vi "2B_Tech Serial Data Recording & DECADE 2.0.vi"() -> ()   [LabVIEW 2014]
uses:
  <vilib>/Instr/_visa.llb/VISA Set IO Buffer Mask.ctl
  <vilib>/Instr/_visa.llb/VISA Flush IO Buffer Mask.ctl
  <vilib>/Platform/TimedLoop/XDataNode/timing_clust.ctl
  <vilib>/Platform/TimedLoop/XDataNode/nitl_modes.ctl
  <vilib>/Platform/TimedLoop/XDataNode/wakeup.ctl
  C:/Program Files (x86)/National Instruments/LabVIEW 2014/examples/Data Communication/Network Streams/Simple Network Streams/support/Network Stream Command.ctl
  <vilib>/Utility/error.llb/whitespace.ctl
  <vilib>/Instr/_visa.llb/VISA Configure Serial Port (Instr).vi
  <vilib>/Utility/tcp.llb/UDP Multicast Write-Only Open.vi
  <vilib>/platform/TimedLoop/XDataNode/XDataNode.xnode
  <vilib>/Platform/TimedLoop/XDataNode/XDNodeRunTimeDep.lvlib
panel:
  out "Default file name":string
  out "error out":errorcluster
  out "Ambient/Cabin":bool
  out "Stop File Write":bool
  in  "timeout (10sec)":u32=3000
  in  "VISA resource name":refnum<visa-resource-name>="ASRL2::INSTR"
  out "Simulate 3 av":dbl
  out "Simulate\nConc":i32
  out "Simulate\nconc":bool
  out "3hr_alm_thresh":i32=80
  out "3hrAvg_Alarm":bool
  out "Inst_Alarm":bool
  out "Inst_alm_thresh":i32=220
  out "Time":string
  in  "Clear Display\nErrors":bool
  out "Read Error Counter\nfrom process loop":u32
  out "CABOZO UDP_ASCII_Out":string
  out "Ozo_array":string[](array[string])
  out "3hr_ozo_avg":dbl
  out "q_size":i32
  out "Data Output":string[](array[string])
  out "UDP packet\nSend status":bool
  out "TWBOZO UDP_ASCII_Out":string
  out "UDP_Out_Error":errorcluster
  out "UDP_Pack_num":u32
  out "Flight Number":string
  out "Number of times \nRead time out":u32
  out "Data Loop count":i32
  out "2B_Serial_error out":errorcluster
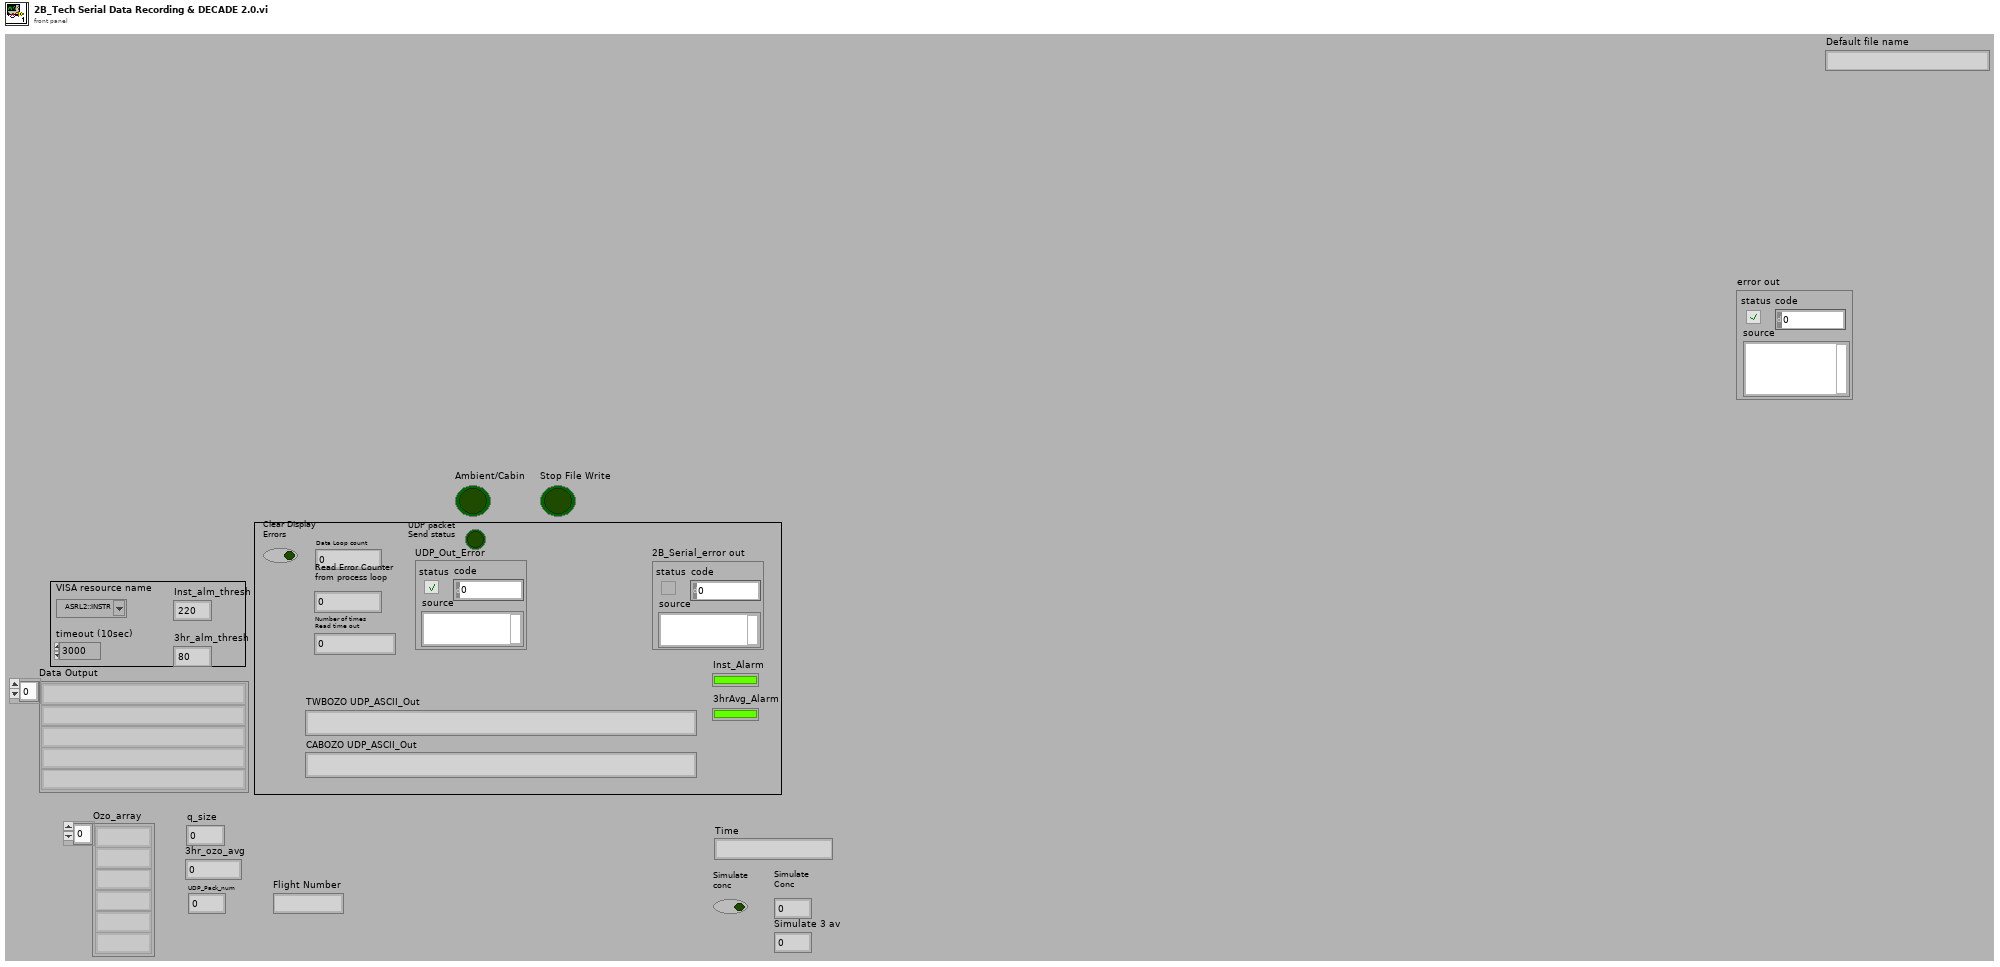
[diagram p1: front panel]
types:
  T1 = typedef "VISA Flush IO Buffer Mask.ctl" = u16
  T2 = typedef "VISA Set IO Buffer Mask.ctl" = u16
  T3 = typedef "Network Stream Command.ctl" = cluster{"Message":string, "Message Data":variant}
  T4 = typedef "XDNodeRunTimeDep.lvlib/timing_clust.ctl" = cluster{"Expected End [f-1]":u64, "Actual End [f-1]":u64, "Finished Late? [f-1]":bool, "Expected End [i-1]":u64, "Actual End [i-1]":u64, "Finished Late? [i-1]":bool, "Expected Start [i]":u64, "Actual Start [i]":u64, "Expected Start [f]":u64, "Actual Start [f]":u64, "Source Name":string, "Structure Name":string, "Period":i64, "Deadline":i64, "Offset":i64, "Start":i64, "Priority":i32, "Timeout":i32, "Mode":T5, "Wakeup Reason":T6, "Error":errorcluster, "Source Type":string, "Secondary Source Type":string, "Global End Time":u64, "Global Start Time":u64, "Frame Duration":u64, "Iteration Duration":u64, "Assigned CPU":i32, "I/O Scan Engine Mode":u32}
  T5 = typedef "XDNodeRunTimeDep.lvlib/nitl_modes.ctl" = enum32{"No Change", "Process missed periods, maintain original phase", "Discard missed periods, maintain original phase", "Process missed periods, ignore original phase", "Discard missed periods, ignore original phase"}
  T6 = typedef "XDNodeRunTimeDep.lvlib/wakeup.ctl" = enum32{"Normal", "Aborted", "Asynchronous wakeup", "Timing source error", "Timed loop error", "Timeout"}
  T7 = enum16{"open", "replace", "create", "open or create", "replace or create", "replace or create with confirmation"}
  T8 = typedef "whitespace.ctl" = u16
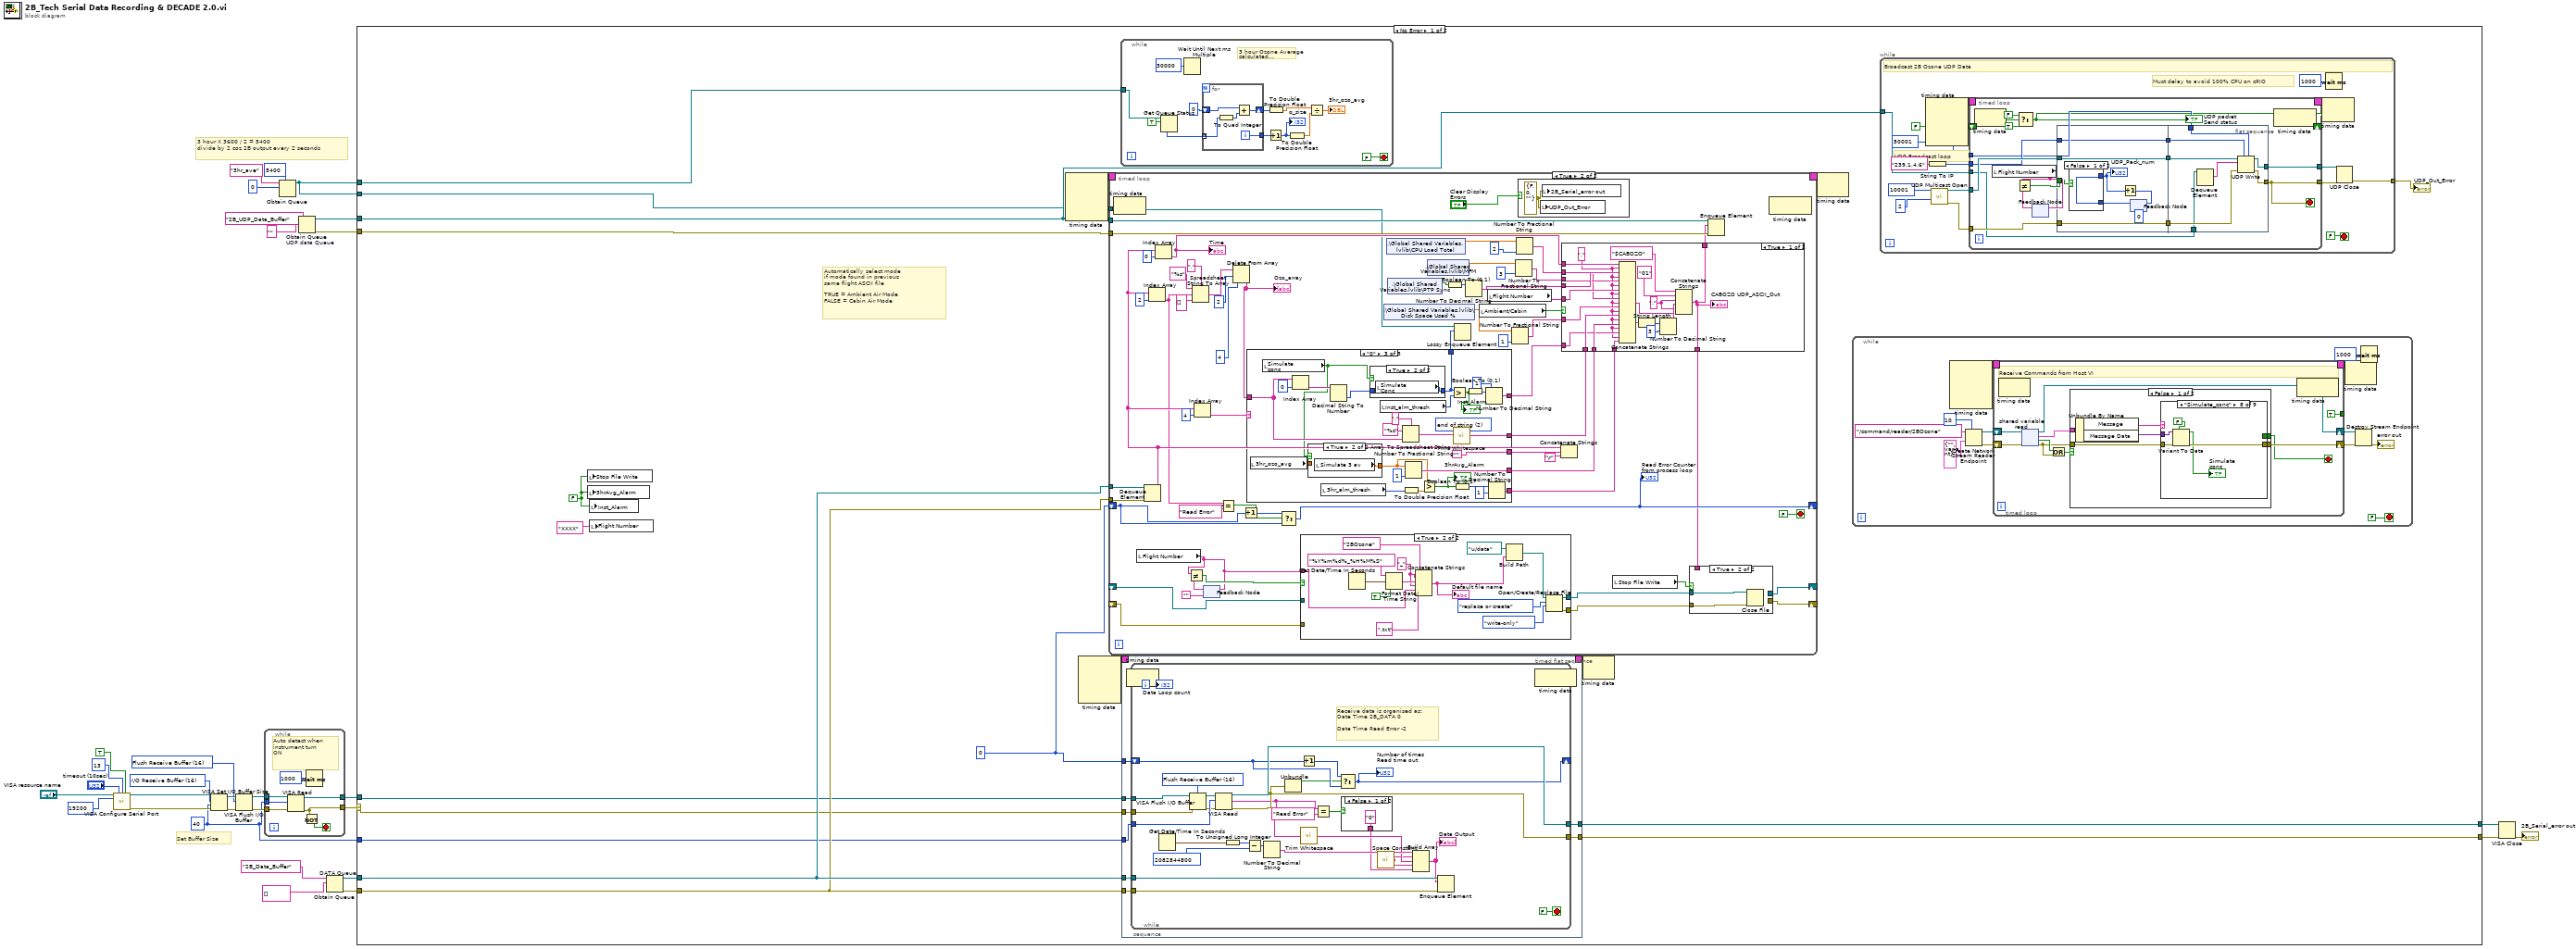
[diagram p0: block diagram]
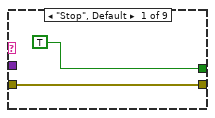
[diagram p2: hidden frame]
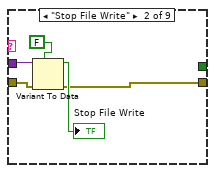
[diagram p3: hidden frame]
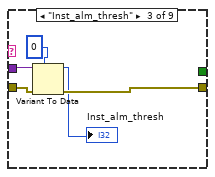
[diagram p4: hidden frame]
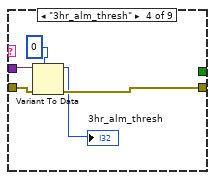
[diagram p5: hidden frame]
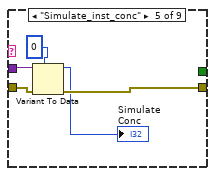
[diagram p6: hidden frame]
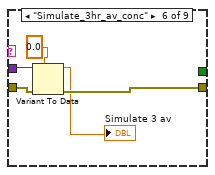
[diagram p7: hidden frame]
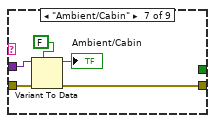
[diagram p8: hidden frame]
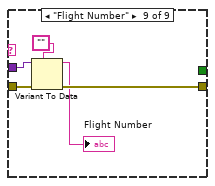
[diagram p9: hidden frame]
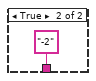
[diagram p11: hidden frame]
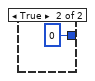
[diagram p12: hidden frame]
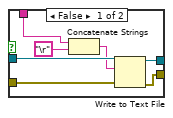
[diagram p13: hidden frame]
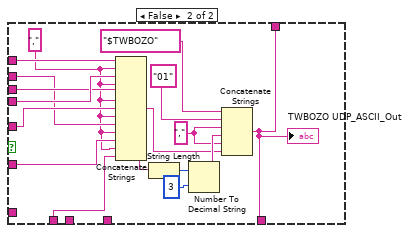
[diagram p16: hidden frame]
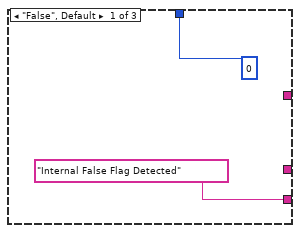
[diagram p17: hidden frame]
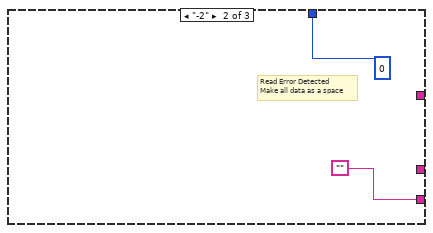
[diagram p18: hidden frame]
diagram:
  w1 = u32 40 ("size (4096)")
  w8 = T1 16 items=["Flush Receive Buffer"=16, "Write Transmit Buffer to Device"=32, "Flush Receive Buffer (No I/O)"=64, "Flush Transmit Buffer"=128] ("Mask")
  w9 = T2 16 items=["I/O Receive Buffer"=16, "I/O Transmit Buffer"=32, "I/O Receive and Transmit Buffer"=48] ("Mask")
  # "Set Buffer Size"
  # "3 hour X 3600 / 2 = 5400\ndivide by 2 coz 2B output every 2 seconds"
  n1 = call-poly "VISA Configure Serial Port"("VISA resource name"="VISA resource name", "timeout (10sec)"="timeout (10sec)", "termination char\n(0xA = '\\n' = LF)"=u8 13 ("termination char\n(0xA = '\\n' = LF)"), "Enable Termination\nChar (T)"=TRUE ("Enable Termination\nChar (T)"), "baud rate (9600)"=u32 19200) -> ("VISA resource name out"=w7:refnum<visa-resource-name>, "error out"=w6:errorcluster)  [unwired: 9 in]
  n2 = VISA Set I/O Buffer Size(VISA resource name=w7, mask (16)=w9, size (4096)=w1, error in (no error)=w6) -> (VISA resource name out=w10:refnum<visa-resource-name>, error out=w11:errorcluster)
  n3 = VISA Flush I/O Buffer(VISA resource name=w10, mask (16)=w8, error in (no error)=w11) -> (VISA resource name out=w5:refnum<visa-resource-name>, error out=w4:errorcluster)
  n4 = while {
    tunnel: w1 -> [w38]
    tunnel: w5 -> [w37]
    tunnel: w4 -> [w36]
    tunnel: [w34] -> w3
    tunnel: [w33] -> w2
    stop <- w35 stop-if-true
    # "Auto detect when\ninstrument turn\nON"
    n5 = VISA Read(VISA resource name=w37, byte count=w38, error in (no error)=w36) -> (VISA resource name out=w33:refnum<visa-resource-name>, error out=w34:errorcluster)  [unwired: 2 out]
    n6 = Not(x=w34) -> (.not. x?=w35:bool)
    n7 = Wait (ms)(milliseconds to wait=u32 1000) -> ()  [unwired: 1 out]
  }
  n8 = Obtain Queue(max queue size (-1, unlimited)=5400, name (unnamed)="3hr_ave", element data type=0 ("index")) -> (queue out=w17:refnum<queue>)  [unwired: 2 in, 2 out]
  n9 = Obtain Queue "UDP data Queue"(name (unnamed)="2B_UDP_Data_Buffer", element data type="") -> (queue out=w23:refnum<queue>, error out=w22:errorcluster)  [unwired: 3 in, 1 out]
  n10 = Obtain Queue "DATA Queue"(name (unnamed)="2B_Data_Buffer", element data type=string[] []) -> (queue out=w27:refnum<queue>, error out=w26:errorcluster)  [unwired: 3 in, 1 out]
  n11 = case shown="No Error" w3 {
    selector: w3 -> [w44 w417]
    tunnel: w2 -> [w45 w418]
    tunnel: [w57 w418] -> w30
    tunnel: [w49 w417] -> w31
    tunnel: w27 -> [w56 _]
    tunnel: w26 -> [w55 _]
    tunnel: w23 -> [w53 _]
    tunnel: w22 -> [w54 _]
    tunnel: w17 -> [w52 _]
    tunnel: w17 -> [w51 _]
    tunnel: w1 -> [w43 _]
    frame No Error {
      w40 = FALSE
      w50 = u32 0
      # "Automatically select mode\nif mode found in previous\nsame flight ASCII file\n\nTRUE = Ambient Air Mode\nFALSE = Cabin Air Mode"
      n12 = local write "Stop File Write"(w40) -> ()
      n13 = local write "3hrAvg_Alarm"(w40) -> ()
      n14 = local write "Inst_Alarm"(w40) -> ()
      n15 = local write "Flight Number"("XXXX" ("Flight Number")) -> ()
      n16 = node-c288() -> (w48:T4)  [unwired: 4 in]
      n17 = node-c288() -> (w42:T4)  [unwired: 4 in]
      n18 = timed-loop {
        timing: w48 -> [_]
        timing-out: [_] -> w47
        tunnel: w56 -> [w315]
        tunnel: w55 -> [w314]
        tunnel: w53 -> [w313]
        tunnel: w54 -> [w312]
        tunnel: w51 -> [w284]
        shift-right: [w288] -> _
        shift-left: w50 -> [w289]
        shift-right: [w277] -> _
        shift-left: _ -> [w273]
        shift-right: [w271] -> _
        shift-left: _ -> [w272]
        stop <- FALSE stop-if-true
        n19 = node-c288() -> ()  [unwired: 1 in, 1 out]
        n20 = local read "Flight Number"() -> (w269:string)
        n21 = Dequeue Element(queue=w315, error in (no error)=w314) -> (element=w297:string[])  [unwired: 1 in, 3 out]
        n22 = Index Array(array=w297, index=2) -> (element=w290:string)
        n23 = Index Array(array=w297, index=0) -> (element=w299:string)
        "Time" <- w299
        n24 = Spreadsheet String To Array(delimiter (Tab)=",", format string="%s", spreadsheet string=w290, array type (2D Dbl)=string[] [] ("Values Array")) -> (array=w304:string[])
        n25 = Index Array(array=w297, index=4) -> (element=w305:string)
        n26 = feedback #1("" ("Flight Number")) -> (w279:string)
        n27 = Not Equal?(x=w269, y=w279) -> (x != y?=w270:bool)
        n28 = feedback-in #1(w269) -> ()
        n29 = Equal?(x=w290, y="Read Error") -> (x = y?=w292:bool)
        n30 = Delete From Array(array=w304, length=2, index=4) -> (array with subset deleted=w301:string[])  [unwired: 1 out]
        "Ozo_array" <- w301
        n31 = Increment(x=w289) -> (x+1=w291:u32)
        n32 = case shown="\"0\"" w305 {
          tunnel: w301 -> [_ _ w401]
          tunnel: [_ _ w404] -> w298
          tunnel: [0 0 w389] -> w283
          tunnel: ["Internal False Flag Detected" "" ""] -> w296
          tunnel: [_ _ w398] -> w294
          tunnel: [_ _ w395] -> w286
          tunnel: [_ _ w391] -> w285
          frame "False", Default {
          }
          frame "-2" {
            # "Read Error Detected\nMake all data as a space"
          }
          frame "0" {
            w405 = T8 2 items=["both", "start of string", "end of string"] ("location (both)")
            n33 = local read "3hr_ozo_avg"() -> (w388:dbl)
            n34 = local read "Simulate\nconc"() -> (w384:bool)
            n35 = Index Array(array=w401, index=0) -> (element=w402:string)
            n36 = case shown="True" w384 {
              tunnel: [w409 w410] -> w387
              tunnel: w388 -> [w409 _]
              frame False {
              }
              frame True {
                n37 = local read "Simulate 3 av"() -> (w410:dbl)
              }
            }
            n38 = local read "3hr_alm_thresh"() -> (w385:i32)
            n39 = Decimal String To Number(string=w402) -> (number=w390:i32)  [unwired: 2 in, 1 out]
            n40 = case shown="True" w384 {
              tunnel: [w411 w412] -> w389
              tunnel: w390 -> [w411 _]
              frame False {
              }
              frame True {
                n41 = local read "Simulate\nConc"() -> (w412:i32)
              }
            }
            n42 = local read "Inst_alm_thresh"() -> (w386:i32)
            n43 = Array To Spreadsheet String(delimiter (Tab)=",", array=w401, 3:"%s" ("format string")) -> (spreadsheet string=w406:string)
            n44 = To Double Precision Float(number=w385) -> (double precision float=w392:dbl)
            n45 = Number To Fractional String(number=w387, precision (6)=i16 1) -> (F-format string=w398:string)  [unwired: 2 in]
            n46 = Greater?(x=w387, y=w392) -> (0:w393:bool)
            "3hrAvg_Alarm" <- w393
            n47 = Greater?(x=w389, y=w386) -> (0:w396:bool)
            "Inst_Alarm" <- w396
            n48 = call <vilib>:"Trim Whitespace.vi"("string"=w406, "location (both)"=w405) -> ("trimmed string"=w404:string)
            n49 = Boolean To (0,1)(Boolean=w393) -> (0, 1=w394:i16)
            n50 = Boolean To (0,1)(Boolean=w396) -> (0, 1=w397:i16)
            n51 = Number To Decimal String(number=w397, width (-)=i16 1) -> (decimal integer string=w395:string)
            n52 = Number To Decimal String(number=w394, width (-)=i16 1) -> (decimal integer string=w391:string)
          }
        }
        n53 = Select(t=w291, s=w292, f=w289) -> (s? t:f=w288:u32)
        "Read Error Counter\nfrom process loop" <- w288
        n54 = case shown="True" w270 {
          tunnel: [w326 w329] -> w275
          tunnel: [w325 w328] -> w274
          tunnel: w273 -> [w326 _]
          tunnel: w272 -> [w325 _]
          tunnel: w269 -> [_ w327]
          frame False {
          }
          frame True {
            w336 = "_" ("string")
            n55 = Get Date/Time In Seconds() -> (seconds since 1Jan1904=w337:timestamp)
            n56 = Format Date/Time String(time format string (%c)="%Y%m%d%_%H%M%S", seconds (now)=w337, UTC format=TRUE) -> (date/time string=w340:string)
            n57 = Concatenate Strings("2BOzone" ("string"), w336, w340, w336, w327, ".txt" ("string")) -> (w334:string)
            "Default file name" <- w334
            n58 = Build Path(base path=path "u:/data", name or relative path=w334) -> (appended path=w330:path)
            n59 = Open/Create/Replace File(file path (use dialog)=w330, operation (0:open)=T7."replace or create", access (0:read/write)=enum16{"read/write", "read-only", "write-only"}."write-only") -> (refnum out=w329:refnum<file>, error out=w328:errorcluster)  [unwired: 3 in, 1 out]
          }
        }
        n60 = shared-variable ".\\Global Shared Variables.lvlib\\Disk Space Used %"() -> (w257:dbl)  [unwired: 1 in, 1 out]
        n61 = shared-variable ".\\Global Shared Variables.lvlib\\CPU Load Total"() -> (w267:dbl)  [unwired: 1 in, 1 out]
        n62 = shared-variable ".\\Global Shared Variables.lvlib\\PTP Sync"() -> (w260:bool)  [unwired: 1 in, 1 out]
        n63 = shared-variable ".\\Global Shared Variables.lvlib\\MFM"() -> (w265:dbl)  [unwired: 1 in, 1 out]
        n64 = Boolean To (0,1)(Boolean=w260) -> (0, 1=w261:i16)
        n65 = Lossy Enqueue Element(queue=w284, element=w283) -> ()  [unwired: 1 in, 4 out]
        n66 = Number To Decimal String(number=w261) -> (decimal integer string=w259:string)  [unwired: 1 in]
        n67 = local read "Ambient/Cabin"() -> (w280:bool)
        n68 = local read "Flight Number"() -> (w281:string)
        n69 = Number To Fractional String(number=w257, precision (6)=i16 1) -> (F-format string=w256:string)  [unwired: 2 in]
        n70 = Number To Fractional String(number=w265, precision (6)=i16 3) -> (F-format string=w262:string)  [unwired: 2 in]
        n71 = Number To Fractional String(number=w267, precision (6)=i16 2) -> (F-format string=w266:string)  [unwired: 2 in]
        n72 = case shown="True" "Clear Display\nErrors" {
          frame False {
          }
          frame True {
            w342 = errorcluster {"status"=FALSE, "code"=0, "source"=""} ("UDP Error Out")
            n73 = local write "UDP_Out_Error"(w342) -> ()
            n74 = local write "2B_Serial_error out"(w342) -> ()
          }
        }
        n75 = Concatenate Strings(w297, w296, "\r") -> ()  [unwired: 1 out]
        n76 = case shown="True" w280 {
          tunnel: [w349 w369] -> w311
          tunnel: w299 -> [w354 w370]
          tunnel: w298 -> [w353 w362]
          tunnel: w266 -> [w345 w365]
          tunnel: w262 -> [w347 w367]
          tunnel: w281 -> [w346 w366]
          tunnel: w294 -> [w352 _]
          tunnel: w286 -> [w351 _]
          tunnel: w285 -> [w350 _]
          tunnel: [w349 w369] -> w268
          tunnel: w259 -> [w348 w368]
          tunnel: w256 -> [w344 w364]
          frame True {
            w343 = ","
            w358 = ","
            n77 = Concatenate Strings(w354, w343, w348, w343, w347, w343, w346, w343, w345, w343, w344, w343, w353, w343, w352, w343, w351, w343, w350) -> (w357:string)
            n78 = String Length(string=w357) -> (length=w361:i32)
            n79 = Number To Decimal String(number=w361, width (-)=i16 3) -> (decimal integer string=w359:string)
            n80 = Concatenate Strings("$CABOZO", "01", w358, w359, w358, w357) -> (w349:string)
            "CABOZO UDP_ASCII_Out" <- w349
          }
          frame False {
            w363 = ","
            w374 = ","
            n81 = Concatenate Strings(w370, w363, w368, w363, w367, w363, w366, w363, w365, w363, w364, w363, w362) -> (w373:string)
            n82 = String Length(string=w373) -> (length=w377:i32)
            n83 = Number To Decimal String(number=w377, width (-)=i16 3) -> (decimal integer string=w375:string)
            n84 = Concatenate Strings("$TWBOZO", "01", w374, w375, w374, w373) -> (w369:string)
            "TWBOZO UDP_ASCII_Out" <- w369
          }
        }
        n85 = local read "Stop File Write"() -> (w276:bool)
        n86 = case shown="True" w276 {
          tunnel: w275 -> [w322 w324]
          tunnel: w274 -> [w321 w323]
          tunnel: [w318 _] -> w277
          tunnel: [w317 _] -> w271
          tunnel: w268 -> [w316 _]
          frame False {
            n87 = Concatenate Strings(w316, "\r") -> (w319:string)
            n88 = Write to Text File(file (use dialog)=w322, text=w319, error in=w321) -> (refnum out=w318:refnum<file>, error out=w317:errorcluster)  [unwired: 2 out]
          }
          frame True {
            n89 = Close File(refnum=w324, error in=w323) -> ()  [unwired: 2 out]
          }
        }
        n90 = Enqueue Element(queue=w313, element=w311, error in (no error)=w312) -> ()  [unwired: 1 in, 3 out]
        n91 = node-c288() -> ()  [unwired: 1 in, 1 out]
      }
      n92 = while {
        tunnel: w52 -> [w188]
        stop <- FALSE stop-if-true
        # "3 hour Ozone Average calculated\nevery 30 seconds"
        n93 = Get Queue Status(queue=w188, return elements? (F)=TRUE) -> (elements=w185:i32[])  [unwired: 1 in, 7 out]
        n94 = Wait Until Next ms Multiple(millisecond multiple=u32 30000) -> ()  [unwired: 1 out]
        n95 = for {
          tunnel: [w200] -> w195
          shift-right: [w199] -> w193
          shift-left: i64 0 -> [w198]
          tunnel: w185 -> [w196] mode=indexing
          i -> [w200]
          n96 = To Quad Integer(1:w196) -> (0:w197:i64)
          n97 = Add(x=w198, y=w197) -> (x+y=w199:i64)
        }
        n98 = Increment(x=w195) -> (x+1=w189:i32)
        "q_size" <- w189
        n99 = To Double Precision Float(number=w193) -> (double precision float=w191:dbl)
        n100 = To Double Precision Float(number=w189) -> (double precision float=w192:dbl)
        n101 = Divide(x=w191, y=w192) -> (x/y=→"3hr_ozo_avg":dbl)
      }
      n102 = timed-sequence {
        timing: w42 -> [_]
        timing-out: [_] -> w41
        tunnel: [w141] -> w57
        tunnel: w56 -> [w140]
        tunnel: w55 -> [w139]
        tunnel: w50 -> [w138]
        tunnel: [w137] -> w49
        tunnel: w45 -> [w136]
        tunnel: w44 -> [w135]
        tunnel: w43 -> [w134]
        n103 = timed-flat-sequence {
          tunnel: [w149] -> w141
          tunnel: w140 -> [w148]
          tunnel: w139 -> [w147]
          tunnel: w138 -> [w146]
          tunnel: [w145] -> w137
          tunnel: w136 -> [w144]
          tunnel: w135 -> [w143]
          tunnel: w134 -> [w142]
          n104 = node-c288() -> ()  [unwired: 1 in, 1 out]
          n105 = while {
            tunnel: [w168] -> w145
            shift-right: [w174] -> _
            shift-left: w146 -> [w175]
            tunnel: [w177] -> w149
            tunnel: w144 -> [w173]
            tunnel: w143 -> [w172]
            tunnel: w148 -> [w171]
            tunnel: w147 -> [w170]
            tunnel: w142 -> [w169]
            i -> [w176]
            stop <- FALSE stop-if-true
            w153 = T1 16 items=["Flush Receive Buffer"=16, "Write Transmit Buffer to Device"=32, "Flush Receive Buffer (No I/O)"=64, "Flush Transmit Buffer"=128] ("Mask")
            # "Receive data is organised as:\nDate Time 2B_DATA 0\n\nDate Time Read Error -2"
            n106 = Get Date/Time In Seconds() -> (seconds since 1Jan1904=w163:timestamp)
            n107 = VISA Flush I/O Buffer(VISA resource name=w173, mask (16)=w153, error in (no error)=w172) -> (VISA resource name out=w154:refnum<visa-resource-name>, error out=w152:errorcluster)
            n108 = VISA Read(VISA resource name=w154, byte count=w169, error in (no error)=w152) -> (VISA resource name out=w177:refnum<visa-resource-name>, read buffer=w151:string, error out=w168:errorcluster)  [unwired: 1 out]
            n109 = To Unsigned Long Integer(number=w163) -> (unsigned 32bit integer=w165:u32)
            n110 = Subtract(x=w165, y=u32 2082844800) -> (x-y=w162:u32)
            n111 = Number To Decimal String(number=w162) -> (decimal integer string=w159:string)  [unwired: 1 in]
            n112 = Unbundle(w168) -> ("status"=w166:bool)  [unwired: 2 out]
            n113 = Increment(x=w175) -> (x+1=w167:u32)
            n114 = call <vilib>:"Trim Whitespace.vi"("string"=w151) -> ("trimmed string"=w158:string)  [unwired: 1 in]
            n115 = Equal?(x=w151, y="Read Error") -> (x = y?=w160:bool)
            n116 = Select(t=w167, s=w166, f=w175) -> (s? t:f=w174:u32)
            "Number of times \nRead time out" <- w174
            n117 = case shown="False" w160 {
              tunnel: ["0" "-2"] -> w156
              frame False {
              }
              frame True {
              }
            }
            n118 = call <vilib>:"Space Constant.vi"() -> ("String"=w157:string)
            n119 = Build Array(w159, w157, w158, w157, w156) -> (w155:string[])
            "Data Output" <- w155
            n120 = Enqueue Element(queue=w171, element=w155, error in (no error)=w170) -> ()  [unwired: 1 in, 3 out]
            "Data Loop count" <- w176
          }
          n121 = node-c288() -> ()  [unwired: 1 in, 1 out]
        }
      }
      n122 = node-c288(w41) -> ()  [unwired: 1 out]
      n123 = node-c288(w47) -> ()  [unwired: 1 out]
      n124 = while {
        stop <- FALSE stop-if-true
        n125 = node-c288() -> (w59:T4)  [unwired: 4 in]
        n126 = Create Network Stream Reader Endpoint(7:10 ("reader buffer size"), 9:T3 {"Message"="", "Message Data"=variant} ("Message Cluster"), 11:"/command/reader/2BOzone" ("reader url")) -> (0:w65:errorcluster, 3:w66:refnum<k21>)  [unwired: 4 in]
        n127 = timed-loop "Host->Target Command Reader" {
          shift-right: [w76] -> w63
          shift-left: w65 -> [w79]
          shift-right: [w77] -> w62
          shift-left: w66 -> [w78]
          tunnel: [TRUE] -> _
          timing: w59 -> [_]
          timing-out: [_] -> w58
          stop <- w70 stop-if-true
          # "Receive Commands from Host VI"
          n128 = node-c288() -> ()  [unwired: 1 in, 1 out]
          n129 = shared-variable-read(w78, w79) -> (w77:refnum<k21>, w72:errorcluster, w74:bool, w75:T3)  [unwired: 1 in]
          n130 = Or(x=w74, y=w72) -> (x .or. y?=w73:bool)
          n131 = case shown="False" w73 {
            selector: w73 -> [_ w130]
            tunnel: w72 -> [w87 w131]
            tunnel: [w86 w131] -> w76
            tunnel: w75 -> [w84 _]
            tunnel: [w85 w130] -> w70
            frame False {
              n132 = Unbundle By Name(w84) -> ("Message"=w83:string, "Message Data"=w82:variant)
              n133 = case shown="\"Simulate_conc\"" w83 {
                tunnel: w87 -> [w89 w94 w99 w104 w109 w114 w119 w124 w129]
                tunnel: [w89 w90 w97 w102 w107 w112 w118 w123 w128] -> w86
                tunnel: w82 -> [_ w93 w98 w103 w108 w113 w117 w122 w127]
                tunnel: [TRUE _ _ _ _ _ _ _ _] -> w85
                frame "Stop", Default {
                }
                frame "Stop File Write" {
                  n134 = Variant To Data(error in=w94, type=FALSE, Variant=w93) -> (data=→"Stop File Write":bool, error out=w90:errorcluster)
                }
                frame "Inst_alm_thresh" {
                  n135 = Variant To Data(error in=w99, type=0, Variant=w98) -> (data=→"Inst_alm_thresh":i32, error out=w97:errorcluster)
                }
                frame "3hr_alm_thresh" {
                  n136 = Variant To Data(error in=w104, type=0, Variant=w103) -> (data=→"3hr_alm_thresh":i32, error out=w102:errorcluster)
                }
                frame "Simulate_inst_conc" {
                  n137 = Variant To Data(error in=w109, type=0, Variant=w108) -> (data=→"Simulate\nConc":i32, error out=w107:errorcluster)
                }
                frame "Simulate_3hr_av_conc" {
                  n138 = Variant To Data(error in=w114, type=0.0, Variant=w113) -> (data=→"Simulate 3 av":dbl, error out=w112:errorcluster)
                }
                frame "Ambient/Cabin" {
                  n139 = Variant To Data(error in=w119, type=FALSE, Variant=w117) -> (data=→"Ambient/Cabin":bool, error out=w118:errorcluster)
                }
                frame "Simulate_conc" {
                  n140 = Variant To Data(error in=w124, type=FALSE, Variant=w122) -> (data=→"Simulate\nconc":bool, error out=w123:errorcluster)
                }
                frame "Flight Number" {
                  n141 = Variant To Data(error in=w129, type="", Variant=w127) -> (data=→"Flight Number":string, error out=w128:errorcluster)
                }
              }
            }
            frame True {
            }
          }
          n142 = node-c288() -> ()  [unwired: 1 in, 1 out]
        }
        n143 = node-c288(w58) -> ()  [unwired: 1 out]
        n144 = Destroy Stream Endpoint(8:w63, 11:w62) -> (0:→"error out":errorcluster)
        n145 = Wait (ms)(milliseconds to wait=u32 1000) -> ()  [unwired: 1 out]
      }
      n146 = while {
        tunnel: w53 -> [w204]
        tunnel: [w203] -> w46
        stop <- FALSE stop-if-true
        # "Must delay to avoid 100% CPU on cRIO"
        # "UDP Broadcast loop"
        # "Broadcast 2B Ozone UDP Data"
        n147 = node-c288() -> (w206:T4)  [unwired: 4 in]
        n148 = String To IP(1:"239.1.4.6" ("name")) -> (0:w208:u32)
        n149 = call-poly <vilib>:"UDP Multicast Open.vi"("time-to-live (1)"=u16 2, "port"=u16 10001) -> ("error out"=w215:errorcluster, "connection ID"=w216:refnum<k16>)  [unwired: 8 in]
        n150 = timed-loop {
          tunnel: w216 -> [w233]
          tunnel: w215 -> [w232]
          tunnel: [w221] -> w211
          shift-right: [w218] -> _
          shift-left: FALSE -> [w226]
          tunnel: [w217] -> w210
          tunnel: w208 -> [w223]
          tunnel: u16 50001 ("port or service name") -> [w222]
          timing: w206 -> [_]
          timing-out: [_] -> w205
          tunnel: w204 -> [w219]
          stop <- w217 stop-if-true
          n151 = node-c288() -> ()  [unwired: 1 in, 1 out]
          n152 = local read "Flight Number"() -> (w220:string)
          n153 = Select(t=FALSE, s=w226, f=TRUE) -> (s? t:f=w218:bool)
          "UDP packet\nSend status" <- w218
          n154 = feedback-in #2(w220) -> ()
          n155 = feedback #2() -> (w228:string)  [unwired: 1 in]
          n156 = Not Equal?(x=w220, y=w228) -> (x != y?=w227:bool)
          n157 = flat-sequence {
            tunnel: w223 -> [w241]
            tunnel: w232 -> [w242]
            tunnel: w233 -> [w243]
            tunnel: [w243] -> w231
            tunnel: [w242] -> w230
            tunnel: [w241] -> w229
            tunnel: w227 -> [w240]
            tunnel: w222 -> [w253]
            tunnel: w231 -> [w252]
            tunnel: w230 -> [w251]
            tunnel: w229 -> [w250]
            tunnel: [w249] -> w221
            tunnel: [w248] -> w217
            tunnel: w219 -> [w246]
            frame #0 {
              n158 = feedback #3(u32 0) -> (w237:u32)
              n159 = case shown="False" w240 {
                tunnel: w237 -> [w244 _]
                tunnel: [w244 u32 0] -> w236
                frame False {
                }
                frame True {
                }
              }
              "UDP_Pack_num" <- w236
              n160 = Increment(x=w236) -> (x+1=w238:u32)
              n161 = feedback-in #3(w238) -> ()
            }
            frame #1 {
              n162 = Dequeue Element(queue=w246) -> (element=w247:string)  [unwired: 2 in, 3 out]
              n163 = UDP Write(address=w250, port or service name=w253, connection ID=w252, data in=w247, 8:w251) -> (error out=w248:errorcluster, 3:w249:refnum<k16>)  [unwired: 1 in]
            }
          }
          n164 = node-c288() -> ()  [unwired: 1 in, 1 out]
        }
        n165 = node-c288(w205) -> ()  [unwired: 1 out]
        n166 = Wait (ms)(milliseconds to wait=u32 1000) -> ()  [unwired: 1 out]
        n167 = UDP Close(connection ID=w211, 8:w210) -> (error out=w203:errorcluster)  [unwired: 1 out]
      }
      "UDP_Out_Error" <- w46
    }
    frame Error {
    }
  }
  n168 = VISA Close(VISA resource name=w30, error in (no error)=w31) -> (error out=→"2B_Serial_error out":errorcluster)
